vi "test noops.vi"() -> (0 "err 538305":errorcluster, 1 "no err":errorcluster, 2 "erro 538305":errorcluster, 3 "error 538305":errorcluster, 4 "er 538305":errorcluster, 5 "warn 538305":errorcluster)   [LabVIEW 2013, in "TBM Tests.lvlib"]
uses:
  TBM Tests.lvlib
  runtime/TBM module execution interface.lvclass
  module configuration/TBM module configuration.lvclass
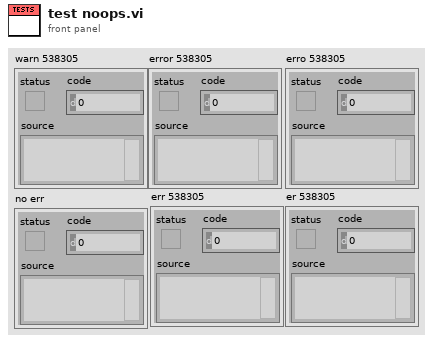
[diagram p1: front panel]
types:
  T1 = typedef "TBM channel.lvclass/data tables.ctl" = cluster{"input data":T2, "processing parameter":T2, "processing result":T2, "output data":T2}
  T2 = typedef "tag bus.lvlib/dictionary table pair.ctl" = cluster{"data dictionary":refnum<class "data dictionary.lvclass">, "data table":T3}
  T3 = typedef "tag bus.lvlib/data table.lvlib/data table.ctl" = cluster{"Double":dbl[], "Single":sgl[], "I64":i64[], "I32":i32[], "I16":i16[], "I8":i8[], "U64":u64[], "U32":u32[], "U16":u16[], "U8":u8[], "Boolean":bool[], "String":string[], "Array of Double":cluster{"DBL Array":dbl[]}[], "Array of Single":cluster{"SGL Array":sgl[]}[], "Array of I64":cluster{"I64 Array":i64[]}[], "Array of I32":cluster{"I32 Array":i32[]}[], "Array of I16":cluster{"I16 Array":i16[]}[], "Array of I8":cluster{"I8 Array":i8[]}[], "Array of U64":cluster{"U64 Array":u64[]}[], "Array of U32":cluster{"U32 Array":u32[]}[], "Array of U16":cluster{"U16 Array":u16[]}[], "Array of U8":cluster{"U8 Array":u8[]}[], "Array of Boolean":cluster{"Boolean Array":bool[]}[], "Array of String":cluster{"String Array":string[]}[]}
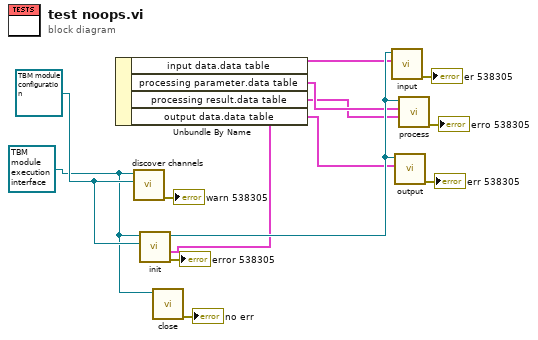
[diagram p0: block diagram]
diagram:
  w13 = refnum<class "TBM module configuration.lvclass"> refnum ("module configuration")
  w10 = refnum<class "TBM module execution interface.lvclass"> refnum ("module")
  n1 = call-dynamic "discover channels.vi"("module configuration"=w13, "module in"=w10) -> ("error out"=→"warn 538305":errorcluster)  [unwired: 7 in, 2 out]
  n2 = call-dynamic "init.vi"("module configuration"=w13, "module in"=w10) -> ("error out"=→"error 538305":errorcluster, "data allocations"=w8:T1, "module out"=w9:refnum<class "TBM module execution interface.lvclass">)  [unwired: 6 in, 1 out]
  n3 = Unbundle By Name(w8) -> ("input data.data table"=w7:T3, "processing parameter.data table"=w6:T3, "processing result.data table"=w5:T3, "output data.data table"=w4:T3)
  n4 = call-dynamic "close.vi"("module in"=w10) -> ("error out"=→"no err":errorcluster)  [unwired: 10 in]
  n5 = call-dynamic "input.vi"("input allocation"=w7, "module in"=w9) -> ("error out"=→"er 538305":errorcluster)  [unwired: 7 in, 2 out]
  n6 = call-dynamic "output.vi"("output data"=w4, "module in"=w9) -> ("error out"=→"err 538305":errorcluster)  [unwired: 7 in, 2 out]
  n7 = call-dynamic "process.vi"("result allocation"=w5, "parameters"=w6, "module in"=w9) -> ("error out"=→"erro 538305":errorcluster)  [unwired: 5 in, 3 out]
